vi "Set Baud Rate.vi"(8 "error in":errorcluster, 11 "Red-y Read Write CFG in":refnum<class "Red-y Read Write CFG.lvclass">) -> (0 "error out":errorcluster, 3 "Red-y Read Write CFG out":refnum<class "Red-y Read Write CFG.lvclass">)   [LabVIEW 2023, in "Red-y Read Write CFG.lvclass"]
uses:
  Red-y Read Write CFG.lvclass
  Red-y Read Write CFG.lvclass/Red-y Read Write CFG.ctl
  Read Write PE Input.ctl
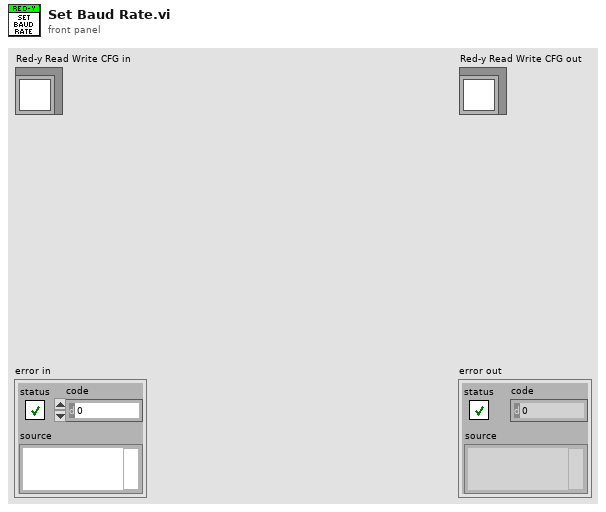
[diagram p1: front panel]
types:
  T1 = typedef "Read Write PE Input.ctl" = cluster{"Action":enum16{"Write", "Read"}, "Register Start Address":u16, "Data (Type)":variant}
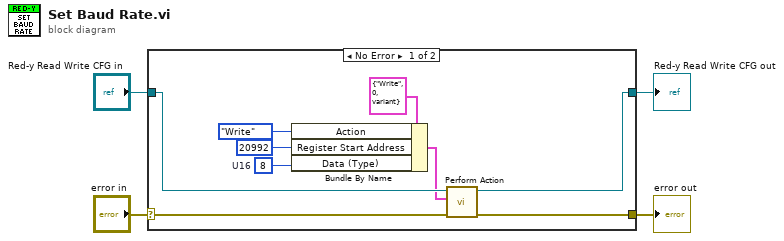
[diagram p0: block diagram]
diagram:
  n1 = case shown="No Error" "error in" {
    selector: "error in" -> [w13 w15]
    tunnel: [w12 w15] -> w3
    tunnel: [w10 w14] -> w1
    tunnel: "Red-y Read Write CFG in" -> [w11 w14]
    frame No Error {
      w5 = u16 8  # U16
      n2 = Bundle By Name(cluster=T1 {"Action"=enum."Write", "Register Start Address"=0, "Data (Type)"=variant}, "Action"=enum16{"Write", "Read"}."Write", "Register Start Address"=u16 20992, "Data (Type)"=w5) -> (w8:T1)
      n3 = call-dynamic "Perform Action.vi"("error in"=w13, "Input"=w8, "Red-y Read Write CFG in"=w11) -> ("error out"=w12:errorcluster, "Red-y Read Write CFG out"=w10:refnum<class "Red-y Read Write CFG.lvclass">)  [unwired: 6 in, 1 out]
    }
    frame Error {
    }
  }
  "error out" <- w3
  "Red-y Read Write CFG out" <- w1
